vi "Chroma 1905x Series Source Cst.vi"(8 "error in (no error)":errorcluster, 11 "VISA resource name":refnum<visa-resource-name>) -> (0 "error out":errorcluster, 3 "VISA resource name out":refnum<visa-resource-name>)   [LabVIEW 2025]
doc: "Chroma\n5 Clock Tower Place Suite 210\nMaynard, MA 01754\nTel: 1 800 253-1230\nTel: 1 877 4 A HIPOT\nFax: 1 978-461-4295\nWebsite: www.chroma.com"
uses:
  <instrlib>/Chrome 19025/Chrome 19025.lvlib
panel:
  # "Capacitance Standar (CST) at\nShort/Open circuit detection Mode"
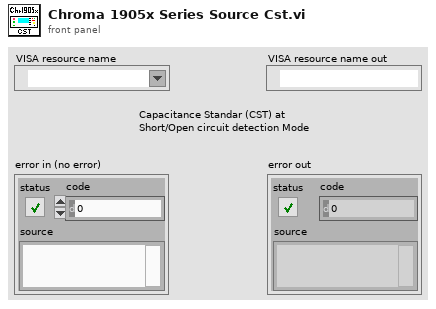
[diagram p1: front panel]
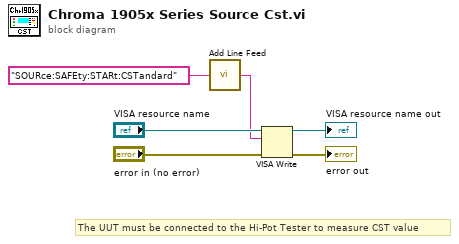
[diagram p0: block diagram]
diagram:
  # "The UUT must be connected to the Hi-Pot Tester to measure CST value"
  n1 = call <instrlib>:"Add Line Feed.vi"("Command string"="SOURce:SAFEty:STARt:CSTandard") -> ("Concatenated string"=w1:string)  [unwired: 4 in]
  n2 = VISA Write(VISA resource name="VISA resource name", write buffer=w1, error in (no error)="error in (no error)") -> (VISA resource name out=→"VISA resource name out":refnum<visa-resource-name>, error out=→"error out":errorcluster)  [unwired: 1 out]
